vi "Lightsensor1Dmodified.vi"(3 "?":bool) -> (0 "Waveform Graph 2":dbl[](graph), 1 "max index(es)":i32, 2 "max value":dbl)   [LabVIEW 2015]
uses:
  <vilib>/Platform/TimedLoop/XDataNode/timing_clust.ctl
  <vilib>/Platform/TimedLoop/XDataNode/nitl_modes.ctl
  <vilib>/Platform/TimedLoop/XDataNode/wakeup.ctl
  <vilib>/imath/engines/lvmath2/RunTimeEngine/NodeEndStatement/NIMS_NodeEndStatement_Output.vi
  <instcachedir>/0/NIMS_NodeEndStatement_Output_53EC0D466D134D7ABD903AC30B43404B.lvgen/NIMS_NodeEndStatement_Output_53EC0D466D134D7ABD903AC30B43404B_010.vi
  <vilib>/imath/engines/lvmath2/RunTimeEngine/ErrorHandling/NIMS_Finalize Error.vi
  <vilib>/platform/TimedLoop/XDataNode/XDataNode.xnode
  <vilib>/Analysis/NI_AALPro.lvlib
  <vilib>/Platform/TimedLoop/XDataNode/XDNodeRunTimeDep.lvlib
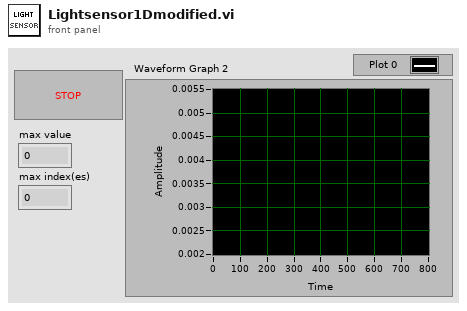
[diagram p1: front panel]
types:
  T1 = typedef "XDNodeRunTimeDep.lvlib/timing_clust.ctl" = cluster{"Expected End [f-1]":u64, "Actual End [f-1]":u64, "Finished Late? [f-1]":bool, "Expected End [i-1]":u64, "Actual End [i-1]":u64, "Finished Late? [i-1]":bool, "Expected Start [i]":u64, "Actual Start [i]":u64, "Expected Start [f]":u64, "Actual Start [f]":u64, "Source Name":string, "Structure Name":string, "Period":i64, "Deadline":i64, "Offset":i64, "Start":i64, "Priority":i32, "Timeout":i32, "Mode":T2, "Wakeup Reason":T3, "Error":errorcluster, "Source Type":string, "Secondary Source Type":string, "Global End Time":u64, "Global Start Time":u64, "Frame Duration":u64, "Iteration Duration":u64, "Assigned CPU":i32, "I/O Scan Engine Mode":u32}
  T2 = typedef "XDNodeRunTimeDep.lvlib/nitl_modes.ctl" = enum32{"No Change", "Process missed periods, maintain original phase", "Discard missed periods, maintain original phase", "Process missed periods, ignore original phase", "Discard missed periods, ignore original phase"}
  T3 = typedef "XDNodeRunTimeDep.lvlib/wakeup.ctl" = enum32{"Normal", "Aborted", "Asynchronous wakeup", "Timing source error", "Timed loop error", "Timeout"}
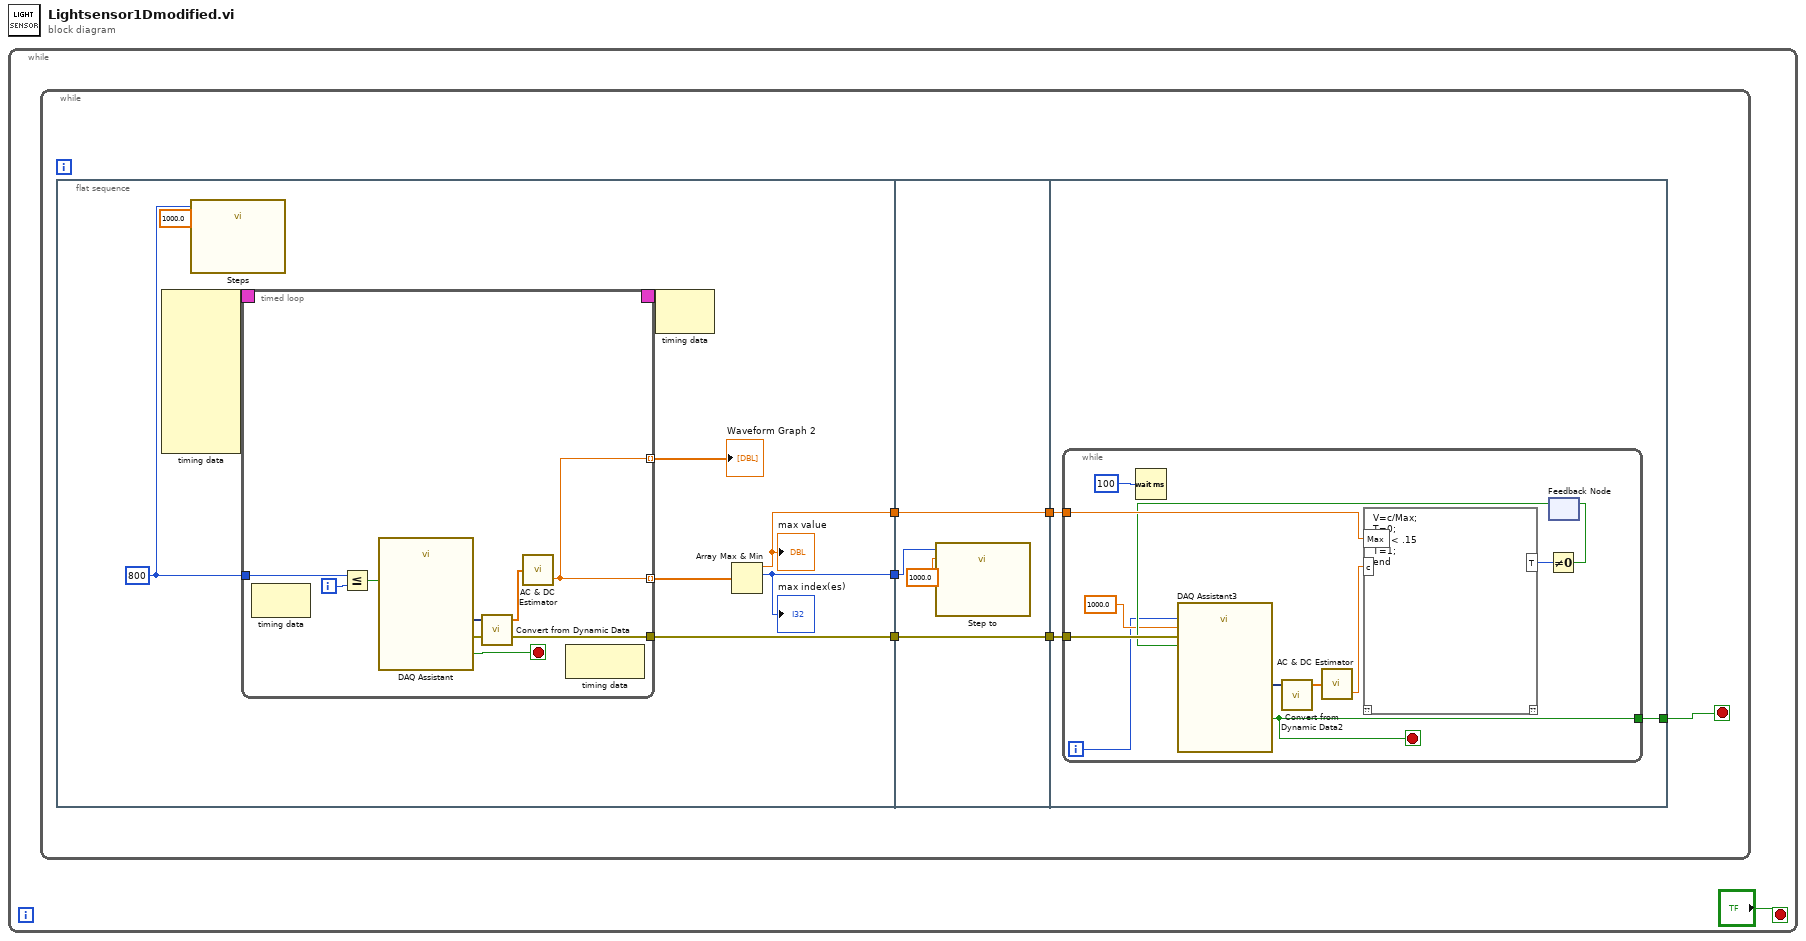
[diagram p0: block diagram]
diagram:
  n1 = while {
    stop <- "?" stop-if-true
    n2 = while {
      stop <- w2 stop-if-true
      n3 = flat-sequence {
        tunnel: [w11] -> w7
        tunnel: [w10] -> w5
        tunnel: [w8] -> w3
        tunnel: w7 -> [w31]
        tunnel: [w30] -> w6
        tunnel: w5 -> [w30]
        tunnel: [w29] -> w4
        tunnel: w3 -> [w29]
        tunnel: w6 -> [w35]
        tunnel: w4 -> [w34]
        tunnel: [w33] -> w2
        frame #0 {
          w9 = 800
          n4 = node-c288() -> (w16:T1)  [unwired: 9 in]
          n5 = call "Steps"("number of samples"=w9, "timeout (s)"=1000.0) -> ()  [unwired: 16 in, 2 out]
          n6 = timed-loop {
            tunnel: [w22] -> w12 mode=indexing
            tunnel: [w22] -> w13 mode=indexing
            timing: w16 -> [_]
            timing-out: [_] -> w15
            tunnel: w9 -> [w18]
            tunnel: [w17] -> w8
            i -> [w19]
            stop <- w20 stop-if-true
            n7 = node-c288() -> ()  [unwired: 1 in, 1 out]
            n8 = Less Or Equal?(x=w18, y=w19) -> (x <= y?=w21:bool)
            n9 = call "DAQ Assistant"("stop (F)"=w21) -> ("data"=w24:dynamicdata, "stopped"=w20:bool, "error out"=w17:errorcluster)  [unwired: 15 in, 1 out]
            n10 = call "Convert from Dynamic Data"("Dynamic Data Type"=w24) -> ("Array"=w23:dbl[])  [unwired: 3 in]
            n11 = call <vilib>:"AC & DC Estimator.vi"("Signal (V)"=w23) -> ("DC estimate (V)"=w22:dbl)  [unwired: 1 out]
            n12 = node-c288() -> ()  [unwired: 1 in, 1 out]
          }
          "Waveform Graph 2" <- w12
          n13 = node-c288(w15) -> ()  [unwired: 1 out]
          n14 = Array Max & Min(array=w13) -> (max value=w10:dbl, max index (indices)=w11:i32)  [unwired: 2 out]
          "max value" <- w10
          "max index(es)" <- w11
        }
        frame #1 {
          n15 = call "Step to"("number of samples"=w31, "timeout (s)"=1000.0) -> ()  [unwired: 16 in, 2 out]
        }
        frame #2 {
          n16 = while {
            tunnel: w35 -> [w43]
            tunnel: w34 -> [w41]
            tunnel: [w38] -> w33
            i -> [w36]
            stop <- w38 stop-if-true
            n17 = Wait (ms)(milliseconds to wait=100) -> ()  [unwired: 1 out]
            n18 = feedback #1() -> (w39:bool)  [unwired: 1 in]
            n19 = call "DAQ Assistant3"("number of samples"=w36, "timeout (s)"=1000.0 ("rate"), "error in"=w41, "stop (F)"=w39) -> ("data"=w47:dynamicdata, "stopped"=w38:bool)  [unwired: 12 in, 2 out]
            n20 = call "Convert from Dynamic Data2"("Dynamic Data Type"=w47) -> ("Array"=w46:dbl[])  [unwired: 3 in]
            n21 = call <vilib>:"AC & DC Estimator.vi"("Signal (V)"=w46) -> ("DC estimate (V)"=w44:dbl)  [unwired: 1 out]
            n22 = mathscript code="V=c/Max;\nT=0;\nif V < .15\nT=1;\nend"("Max"=w43, "c"=w44) -> ("T"=w45:i32)  [unwired: 1 in, 1 out]
            n23 = Not Equal To 0?(x=w45) -> (x != 0?=w40:bool)
            n24 = feedback-in #1(w40) -> ()
          }
        }
      }
    }
  }
